vi "read_ini.vi"() -> (2 "Spectrometer out":refnum<class "Spectrometer.lvclass">, 3 "Camera out":refnum<class "Camera.lvclass">, 4 "DAQ out":refnum<class "DAQ.lvclass">, 6 "Galvo out":refnum<class "Galvonometer.lvclass">, 10 "Proc out":refnum<class "ConfigProc.lvclass">, 14 "PC out":refnum<class "PC.lvclass">, 15 "error out":errorcluster)   [LabVIEW 2017]
doc: "Illustrates how to read a configuration settings file. Run Write Configuration (INI) File.vi. Then run this VI."
uses:
  classes/HardwareObjects/PC/PC.lvclass
  classes/HardwareObjects/Galvonometer/Galvonometer.lvclass
  classes/HardwareObjects/DAQ/DAQ.lvclass
  classes/HardwareObjects/Camera/Camera.lvclass
  classes/HardwareObjects/Spectrometer/Spectrometer.lvclass
  classes/SoftwareObjects/ConfigProc/ConfigProc.lvclass
  classes/HardwareObjects/Spectrometer/Spectrometer.lvclass/Spectrometer.ctl
  classes/HardwareObjects/Camera/Camera.lvclass/Camera.ctl
  classes/HardwareObjects/DAQ/DAQ.lvclass/DAQ.ctl
  classes/HardwareObjects/Galvonometer/Galvonometer.lvclass/Galvonometer.ctl
  classes/HardwareObjects/PC/PC.lvclass/PC.ctl
  classes/SoftwareObjects/ConfigProc/ConfigProc.lvclass/ConfigProc.ctl
  classes/HardwareObjects/Spectrometer/Write Bandwidth (nm).vi
  classes/HardwareObjects/Spectrometer/Write Center wavelength (nm).vi
  classes/HardwareObjects/Spectrometer/Write Make Model.vi
  classes/HardwareObjects/Spectrometer/Write Scan depth (mm).vi
  classes/HardwareObjects/Camera/Write Bit Depth.vi
  classes/HardwareObjects/Camera/Write Camera Dimensions.vi
  classes/HardwareObjects/Camera/Write Data Representation.vi
  classes/HardwareObjects/Camera/Write Duty Cycle.vi
  classes/HardwareObjects/Camera/Write Make, Model.vi
  classes/HardwareObjects/Camera/Write Max Frequency (kHz).vi
  classes/HardwareObjects/Camera/Write Return Time (us).vi
  classes/HardwareObjects/DAQ/Write Camera Counter.vi
  classes/HardwareObjects/DAQ/Write Camera Counter Output Terminal.vi
  classes/HardwareObjects/DAQ/Write Galvo Analog Output Channel(s).vi
  classes/HardwareObjects/DAQ/Write Galvo Counter.vi
  classes/HardwareObjects/DAQ/Write Galvo Counter Terminal.vi
  classes/HardwareObjects/DAQ/Write Master Counter.vi
  classes/HardwareObjects/DAQ/Write Master Counter Terminal.vi
  classes/HardwareObjects/Galvonometer/Write Make Model.vi
  classes/HardwareObjects/Galvonometer/Write Max Scan Angle (degrees).vi
  classes/HardwareObjects/Galvonometer/Write Output Scale Factor (V_degrees).vi
  classes/HardwareObjects/PC/Write Max Number of Cores.vi
  classes/HardwareObjects/PC/Write Path to DLL.vi
  classes/SoftwareObjects/ConfigProc/Write Blur Coefficient.vi
  classes/SoftwareObjects/ConfigProc/Write Blur Int.vi
  classes/SoftwareObjects/ConfigProc/Write Cores.vi
  classes/SoftwareObjects/ConfigProc/Write Interpolation.vi
  classes/SoftwareObjects/ConfigProc/Write Magnification.vi
  classes/SoftwareObjects/ConfigProc/Write Power.vi
  classes/SoftwareObjects/ConfigProc/Write Soften.vi
  classes/HardwareObjects/Spectrometer/Read Bandwidth (nm).vi
  classes/HardwareObjects/Spectrometer/Read Center wavelength (nm).vi
  classes/HardwareObjects/Spectrometer/Read Make Model.vi
  classes/HardwareObjects/Spectrometer/Read Scan depth (mm).vi
  <vilib>/Utility/config.llb/Read Key (Double).vi
  <vilib>/Utility/config.llb/Read Key (String).vi
  <vilib>/Utility/config.llb/NI_LVConfig.lvlib
panel:
  in  "Proc in":refnum<class "ConfigProc.lvclass">
  out "Spectrometer properties":T1
  in  "Spectrometer":refnum<class "Spectrometer.lvclass">
  in  "Def Camera":refnum<class "Camera.lvclass">
  in  "Def DAQ":refnum<class "DAQ.lvclass">
  in  "Def Galvo X":refnum<class "Galvonometer.lvclass">
  in  "Def PC":refnum<class "PC.lvclass">
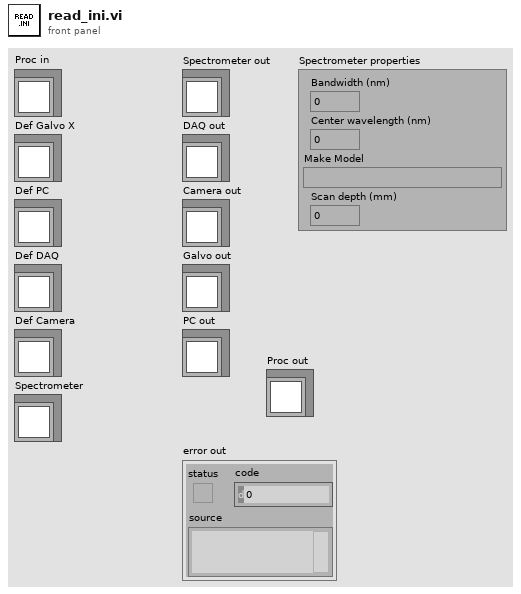
[diagram p1: front panel]
types:
  T1 = cluster{"Bandwidth (nm)":dbl, "Center wavelength (nm)":dbl, "Make Model":string, "Scan depth (mm)":dbl}
  T2 = typedef "NI_LVConfig.lvlib/Config Data RefNum.ctl" = refnum<k1>
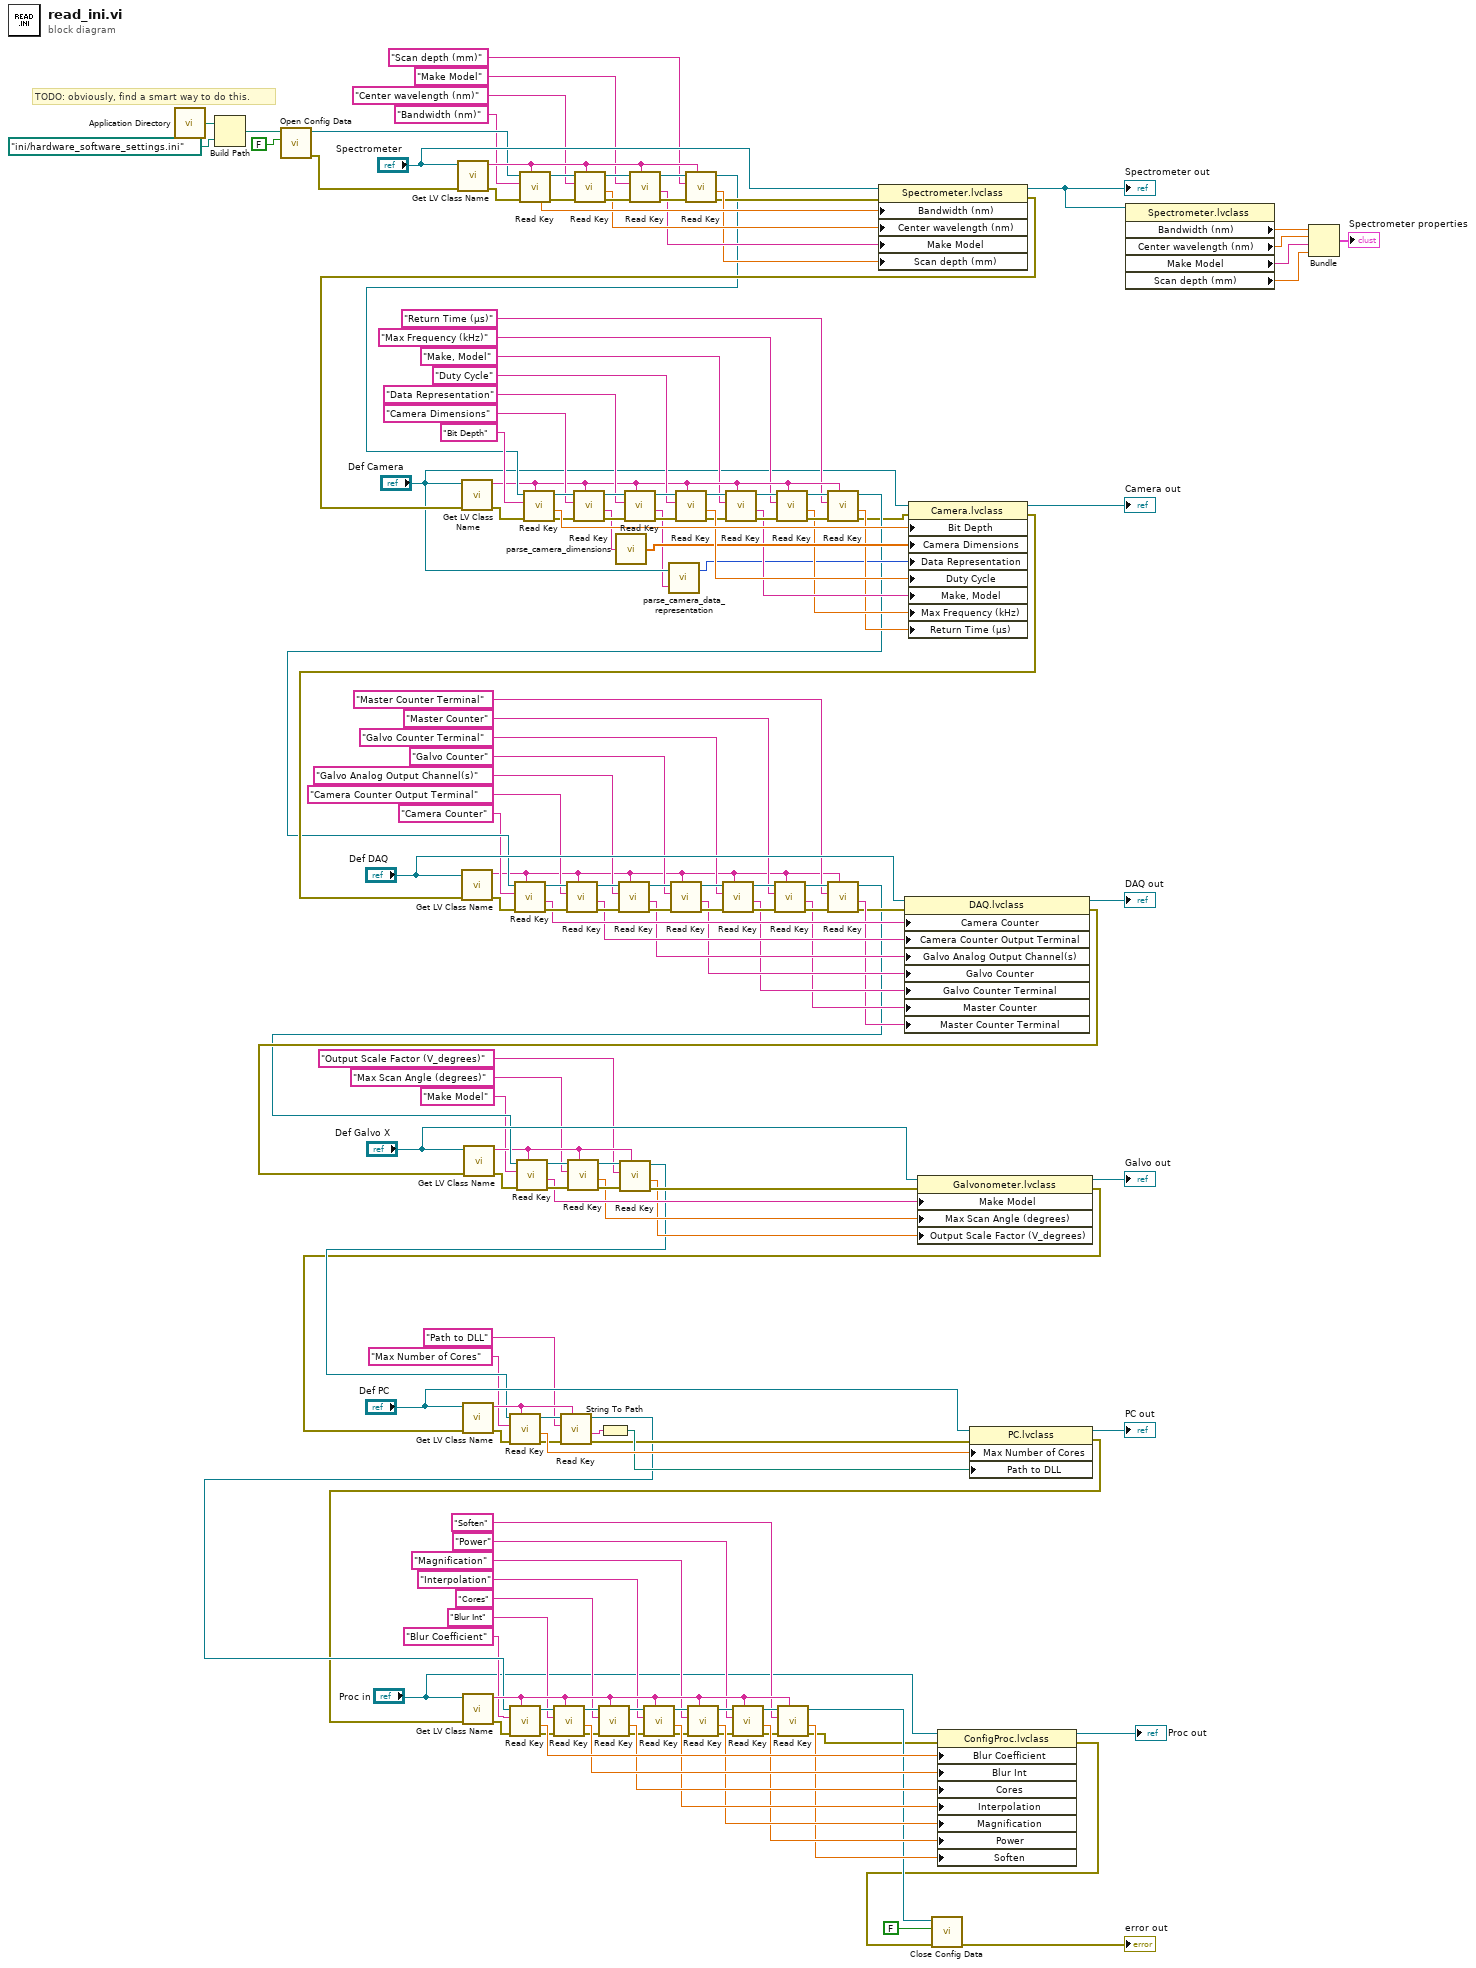
[diagram p0: block diagram]
diagram:
  # "TODO: obviously, find a smart way to do this."
  n1 = call <vilib>:"Application Directory.vi"() -> ("Application Directory"=w159:path)
  n2 = Build Path(base path=w159, name or relative path=path "ini/hardware_software_settings.ini" ("default name")) -> (appended path=w158:path)
  n3 = call <vilib>:"Open Config Data.vi"("create file if necessary (T)"=FALSE ("create file if necessary? (T)"), "configuration file path"=w158) -> ("error out"=w155:errorcluster, "refnum"=w152:T2)  [unwired: 7 in, 1 out]
  n4 = call <vilib>:"Get LV Class Name.vi"("error in (no error)"=w155, "object"="Spectrometer") -> ("error out"=w154:errorcluster, "class name"=w153:string)  [unwired: 8 in]
  n5 = call-poly <vilib>:"Read Key.vi"("section"=w153, "error in (no error)"=w154, "key"="Bandwidth (nm)", "refnum"=w152) -> ("error out"=w147:errorcluster, "value"=w157:dbl, "refnum out"=w150:T2)  [unwired: 1 in, 4 out]
  n6 = call-poly <vilib>:"Read Key.vi"("section"=w153, "error in (no error)"=w147, "key"="Center wavelength (nm)", "refnum"=w150) -> ("error out"=w146:errorcluster, "value"=w141:dbl, "refnum out"=w149:T2)  [unwired: 1 in, 4 out]
  n7 = call-poly <vilib>:"Read Key.vi"("section"=w153, "error in (no error)"=w146, "key"="Make Model", "refnum"=w149) -> ("error out"=w145:errorcluster, "value"=w140:string, "refnum out"=w148:T2)  [unwired: 2 in, 3 out]
  n8 = call-poly <vilib>:"Read Key.vi"("section"=w153, "error in (no error)"=w145, "key"="Scan depth (mm)", "refnum"=w148) -> ("error out"=w138:errorcluster, "value"=w139:dbl, "refnum out"=w123:T2)  [unwired: 1 in, 4 out]
  n9 = property class="Spectrometer.lvclass"(reference="Spectrometer", error in=w138, "Bandwidth (nm)"=w157, "Center wavelength (nm)"=w141, "Make Model"=w140, "Scan depth (mm)"=w139) -> (reference out=w8:refnum<class "Spectrometer.lvclass">, error out=w166:errorcluster)
  "Spectrometer out" <- w8
  n10 = call <vilib>:"Get LV Class Name.vi"("error in (no error)"=w166, "object"="Def Camera") -> ("error out"=w136:errorcluster, "class name"=w119:string)  [unwired: 8 in]
  n11 = call-poly <vilib>:"Read Key.vi"("section"=w119, "error in (no error)"=w136, "key"="Bit Depth", "refnum"=w123) -> ("error out"=w131:errorcluster, "value"=w137:dbl, "refnum out"=w134:T2)  [unwired: 1 in, 4 out]
  n12 = call-poly <vilib>:"Read Key.vi"("section"=w119, "error in (no error)"=w131, "key"="Camera Dimensions", "refnum"=w134) -> ("error out"=w130:errorcluster, "value"=w118:string, "refnum out"=w133:T2)  [unwired: 2 in, 3 out]
  n13 = call "parse_camera_dimensions.vi"("String"=w118) -> ("Camera Dimensions Out"=w117:dbl[])
  n14 = call-poly <vilib>:"Read Key.vi"("section"=w119, "error in (no error)"=w130, "key"="Data Representation", "refnum"=w133) -> ("error out"=w129:errorcluster, "value"=w106:string, "refnum out"=w132:T2)  [unwired: 2 in, 3 out]
  n15 = call "parse_camera_data_representation.vi"("String"=w106, "Def Camera"="Def Camera") -> ("Data Representation Out"=w105:enum16{"U8", "I8", "U16", "I16"})  [unwired: 1 out]
  n16 = call-poly <vilib>:"Read Key.vi"("section"=w119, "error in (no error)"=w129, "key"="Duty Cycle", "refnum"=w132) -> ("error out"=w113:errorcluster, "value"=w125:dbl, "refnum out"=w122:T2)  [unwired: 1 in, 4 out]
  n17 = call-poly <vilib>:"Read Key.vi"("section"=w119, "error in (no error)"=w113, "key"="Make, Model", "refnum"=w122) -> ("error out"=w112:errorcluster, "value"=w110:string, "refnum out"=w121:T2)  [unwired: 2 in, 3 out]
  n18 = call-poly <vilib>:"Read Key.vi"("section"=w119, "error in (no error)"=w112, "key"="Max Frequency (kHz)", "refnum"=w121) -> ("error out"=w111:errorcluster, "value"=w109:dbl, "refnum out"=w120:T2)  [unwired: 1 in, 4 out]
  n19 = call-poly <vilib>:"Read Key.vi"("section"=w119, "error in (no error)"=w111, "key"="Return Time (µs)", "refnum"=w120) -> ("error out"=w75:errorcluster, "value"=w108:dbl, "refnum out"=w103:T2)  [unwired: 1 in, 4 out]
  n20 = property class="Camera.lvclass"(reference="Def Camera", error in=w75, "Bit Depth"=w137, "Camera Dimensions"=w117, "Data Representation"=w105, "Duty Cycle"=w125, "Make, Model"=w110, "Max Frequency (kHz)"=w109, "Return Time (µs)"=w108) -> (reference out=→"Camera out":refnum<class "Camera.lvclass">, error out=w165:errorcluster)
  n21 = call <vilib>:"Get LV Class Name.vi"("error in (no error)"=w165, "object"="Def DAQ") -> ("error out"=w76:errorcluster, "class name"=w9:string)  [unwired: 8 in]
  n22 = call-poly <vilib>:"Read Key.vi"("section"=w9, "error in (no error)"=w76, "key"="Camera Counter", "refnum"=w103) -> ("error out"=w96:errorcluster, "value"=w83:string, "refnum out"=w102:T2)  [unwired: 2 in, 3 out]
  n23 = call-poly <vilib>:"Read Key.vi"("section"=w9, "error in (no error)"=w96, "key"="Camera Counter Output Terminal", "refnum"=w102) -> ("error out"=w95:errorcluster, "value"=w82:string, "refnum out"=w101:T2)  [unwired: 2 in, 3 out]
  n24 = call-poly <vilib>:"Read Key.vi"("section"=w9, "error in (no error)"=w95, "key"="Galvo Analog Output Channel(s)", "refnum"=w101) -> ("error out"=w94:errorcluster, "value"=w81:string, "refnum out"=w100:T2)  [unwired: 2 in, 3 out]
  n25 = call-poly <vilib>:"Read Key.vi"("section"=w9, "error in (no error)"=w94, "key"="Galvo Counter", "refnum"=w100) -> ("error out"=w93:errorcluster, "value"=w80:string, "refnum out"=w99:T2)  [unwired: 2 in, 3 out]
  n26 = call-poly <vilib>:"Read Key.vi"("section"=w9, "error in (no error)"=w93, "key"="Galvo Counter Terminal", "refnum"=w99) -> ("error out"=w92:errorcluster, "value"=w79:string, "refnum out"=w98:T2)  [unwired: 2 in, 3 out]
  n27 = call-poly <vilib>:"Read Key.vi"("section"=w9, "error in (no error)"=w92, "key"="Master Counter", "refnum"=w98) -> ("error out"=w91:errorcluster, "value"=w78:string, "refnum out"=w97:T2)  [unwired: 2 in, 3 out]
  n28 = call-poly <vilib>:"Read Key.vi"("section"=w9, "error in (no error)"=w91, "key"="Master Counter Terminal", "refnum"=w97) -> ("error out"=w72:errorcluster, "value"=w77:string, "refnum out"=w71:T2)  [unwired: 2 in, 3 out]
  n29 = property class="DAQ.lvclass"(reference="Def DAQ", error in=w72, "Camera Counter"=w83, "Camera Counter Output Terminal"=w82, "Galvo Analog Output Channel(s)"=w81, "Galvo Counter"=w80, "Galvo Counter Terminal"=w79, "Master Counter"=w78, "Master Counter Terminal"=w77) -> (reference out=→"DAQ out":refnum<class "DAQ.lvclass">, error out=w164:errorcluster)
  n30 = call <vilib>:"Get LV Class Name.vi"("error in (no error)"=w164, "object"="Def Galvo X") -> ("error out"=w73:errorcluster, "class name"=w70:string)  [unwired: 8 in]
  n31 = call-poly <vilib>:"Read Key.vi"("section"=w70, "error in (no error)"=w73, "key"="Make Model", "refnum"=w71) -> ("error out"=w67:errorcluster, "value"=w61:string, "refnum out"=w69:T2)  [unwired: 2 in, 3 out]
  n32 = call-poly <vilib>:"Read Key.vi"("section"=w70, "error in (no error)"=w67, "key"="Max Scan Angle (degrees)", "refnum"=w69) -> ("error out"=w66:errorcluster, "value"=w60:dbl, "refnum out"=w68:T2)  [unwired: 1 in, 4 out]
  n33 = call-poly <vilib>:"Read Key.vi"("section"=w70, "error in (no error)"=w66, "key"="Output Scale Factor (V_degrees)", "refnum"=w68) -> ("error out"=w65:errorcluster, "value"=w59:dbl, "refnum out"=w54:T2)  [unwired: 1 in, 4 out]
  n34 = property class="Galvonometer.lvclass"(reference="Def Galvo X", error in=w65, "Make Model"=w61, "Max Scan Angle (degrees)"=w60, "Output Scale Factor (V_degrees)"=w59) -> (reference out=→"Galvo out":refnum<class "Galvonometer.lvclass">, error out=w45:errorcluster)
  n35 = call <vilib>:"Get LV Class Name.vi"("error in (no error)"=w45, "object"="Def PC") -> ("error out"=w44:errorcluster, "class name"=w55:string)  [unwired: 8 in]
  n36 = call-poly <vilib>:"Read Key.vi"("section"=w55, "error in (no error)"=w44, "key"="Max Number of Cores", "refnum"=w54) -> ("error out"=w47:errorcluster, "value"=w49:dbl, "refnum out"=w53:T2)  [unwired: 1 in, 4 out]
  n37 = call-poly <vilib>:"Read Key.vi"("section"=w55, "error in (no error)"=w47, "key"="Path to DLL", "refnum"=w53) -> ("error out"=w46:errorcluster, "value"=w50:string, "refnum out"=w27:T2)  [unwired: 2 in, 3 out]
  n38 = String To Path(string=w50) -> (path=w48:path)
  n39 = property class="PC.lvclass"(reference="Def PC", error in=w46, "Max Number of Cores"=w49, "Path to DLL"=w48) -> (reference out=→"PC out":refnum<class "PC.lvclass">, error out=w10:errorcluster)
  n40 = call <vilib>:"Get LV Class Name.vi"("error in (no error)"=w10, "object"="Proc in") -> ("error out"=w37:errorcluster, "class name"=w36:string)  [unwired: 8 in]
  n41 = call-poly <vilib>:"Read Key.vi"("section"=w36, "error in (no error)"=w37, "key"="Blur Coefficient", "refnum"=w27) -> ("error out"=w25:errorcluster, "value"=w35:dbl, "refnum out"=w43:T2)  [unwired: 1 in, 4 out]
  n42 = call-poly <vilib>:"Read Key.vi"("section"=w36, "error in (no error)"=w25, "key"="Blur Int", "refnum"=w43) -> ("error out"=w24:errorcluster, "value"=w34:dbl, "refnum out"=w42:T2)  [unwired: 1 in, 4 out]
  n43 = call-poly <vilib>:"Read Key.vi"("section"=w36, "error in (no error)"=w24, "key"="Cores", "refnum"=w42) -> ("error out"=w23:errorcluster, "value"=w33:dbl, "refnum out"=w41:T2)  [unwired: 1 in, 4 out]
  n44 = call-poly <vilib>:"Read Key.vi"("section"=w36, "error in (no error)"=w23, "key"="Interpolation", "refnum"=w41) -> ("error out"=w22:errorcluster, "value"=w32:dbl, "refnum out"=w40:T2)  [unwired: 1 in, 4 out]
  n45 = call-poly <vilib>:"Read Key.vi"("section"=w36, "error in (no error)"=w22, "key"="Magnification", "refnum"=w40) -> ("error out"=w21:errorcluster, "value"=w31:dbl, "refnum out"=w39:T2)  [unwired: 1 in, 4 out]
  n46 = call-poly <vilib>:"Read Key.vi"("section"=w36, "error in (no error)"=w21, "key"="Power", "refnum"=w39) -> ("error out"=w20:errorcluster, "value"=w30:dbl, "refnum out"=w38:T2)  [unwired: 1 in, 4 out]
  n47 = call-poly <vilib>:"Read Key.vi"("section"=w36, "error in (no error)"=w20, "key"="Soften", "refnum"=w38) -> ("error out"=w19:errorcluster, "value"=w29:dbl, "refnum out"=w26:T2)  [unwired: 1 in, 4 out]
  n48 = property class="ConfigProc.lvclass"(reference="Proc in", error in=w19, "Blur Coefficient"=w35, "Blur Int"=w34, "Cores"=w33, "Interpolation"=w32, "Magnification"=w31, "Power"=w30, "Soften"=w29) -> (reference out=→"Proc out":refnum<class "ConfigProc.lvclass">, error out=w18:errorcluster)
  n49 = call <vilib>:"Close Config Data.vi"("error in (no error)"=w18, "write file if changed (T)"=FALSE ("write configuration file? (T)"), "refnum"=w26) -> ("error out"=→"error out":errorcluster)  [unwired: 8 out]
  n50 = property class="Spectrometer.lvclass"(reference=w8) -> ("Bandwidth (nm)"=w7:dbl, "Center wavelength (nm)"=w6:dbl, "Make Model"=w5:string, "Scan depth (mm)"=w4:dbl)  [unwired: 1 in, 2 out]
  n51 = Bundle("Bandwidth (nm)"=w7, "Center wavelength (nm)"=w6, "Make Model"=w5, "Scan depth (mm)"=w4) -> (→"Spectrometer properties":T1)  [unwired: 1 in]
